vi "Thermal Waveforms.vi"(10 "Log Read Data":cluster{refnum<class "RDS State.lvclass">[]}[](array[cluster]), 11 "Header":T1) -> (2 "Log Data Out":cluster{refnum<class "RDS State.lvclass">[]}[](array[cluster]), 3 "Header Out":T1, 5 "Thermal WFs":waveform(dbl)[](array[waveform]))   [LabVIEW 2015, in "Log Waveform Processors.lvlib"]
uses:
  Log Waveform Processors.lvlib
  RDS State Tracker/RDS State/RDS State.lvclass
  Actors/RDS Logger Actor/RDS Logger Actor/RDS Logger Actor/Logger Header.ctl
  RDS State Tracker/RDS State/RDS State.lvclass/RDS State.ctl
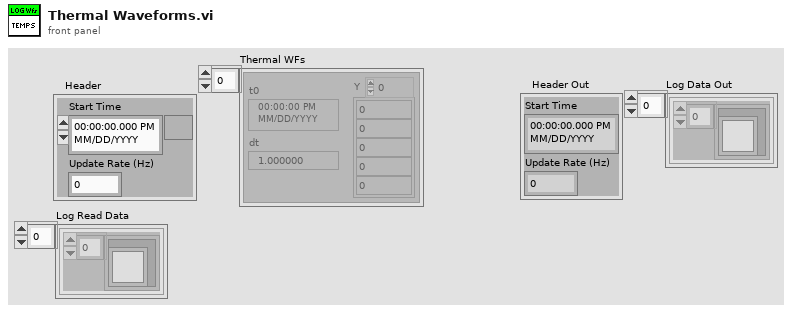
[diagram p1: front panel]
types:
  T1 = typedef "Log Waveform Processors.lvlib/Logger Header.ctl" = cluster{"Start Time":timestamp, "Update Rate (Hz)":dbl}
  T2 = typedef "RDS Instrument Library.lvlib/Battery Data.ctl" = cluster{"Battery Status":T3, "Pack Voltage":sgl, "Pack Current":sgl, "Pack Capacity":sgl, "Max Cell Temp":sgl, "Min Cell Temp":sgl, "Max Cell Voltage":sgl, "Min Cell Voltage":sgl}
  T3 = typedef "RDS Instrument Library.lvlib/Battery Status.ctl" = enum16{"Pack Normal", "Alarm: Cell temp too high", "Alarm: Pack voltage too high", "Warn: Pack voltage too high ", "Alarm: Pack voltage too low", "Warn: Pack voltage low", "Alarm Pack current too high", "Warn: Pack current too high ", "Fault: Pack to chassis connection detected", "Fault: Pack to cell connection error", "Fautl: System error"}
  T4 = typedef "RDS Instrument Library.lvlib/Compass Data.ctl" = cluster{"Compass Heading":sgl, "pitch Angle":sgl, "roll Angle":sgl, "Temperature":sgl, "Depth":sgl, "Magnetic Field":sgl, "Magnetic Field X":sgl, "Magnetic Field Y":sgl, "Magnetic Field Z":sgl, "Acceleration":sgl, "Acceleration X":sgl, "Acceleration Y":sgl, "Gyro":sgl, "Gyro X":sgl, "Acceleration Z":sgl, "Gyro Y":sgl, "Raw Heading":sgl}
  T5 = typedef "RDS Child Messages.lvlib/MCB Motor Status.ctl" = cluster{"Motor Power":i16, "Motor Command":i16, "Battery Volts":sgl, "Battery Amps":sgl, "Motor Amps":sgl, "MCU Temp":i16, "Heatsink Temp":i16, "Fault Flags":u16, "StatusFlags":u16}
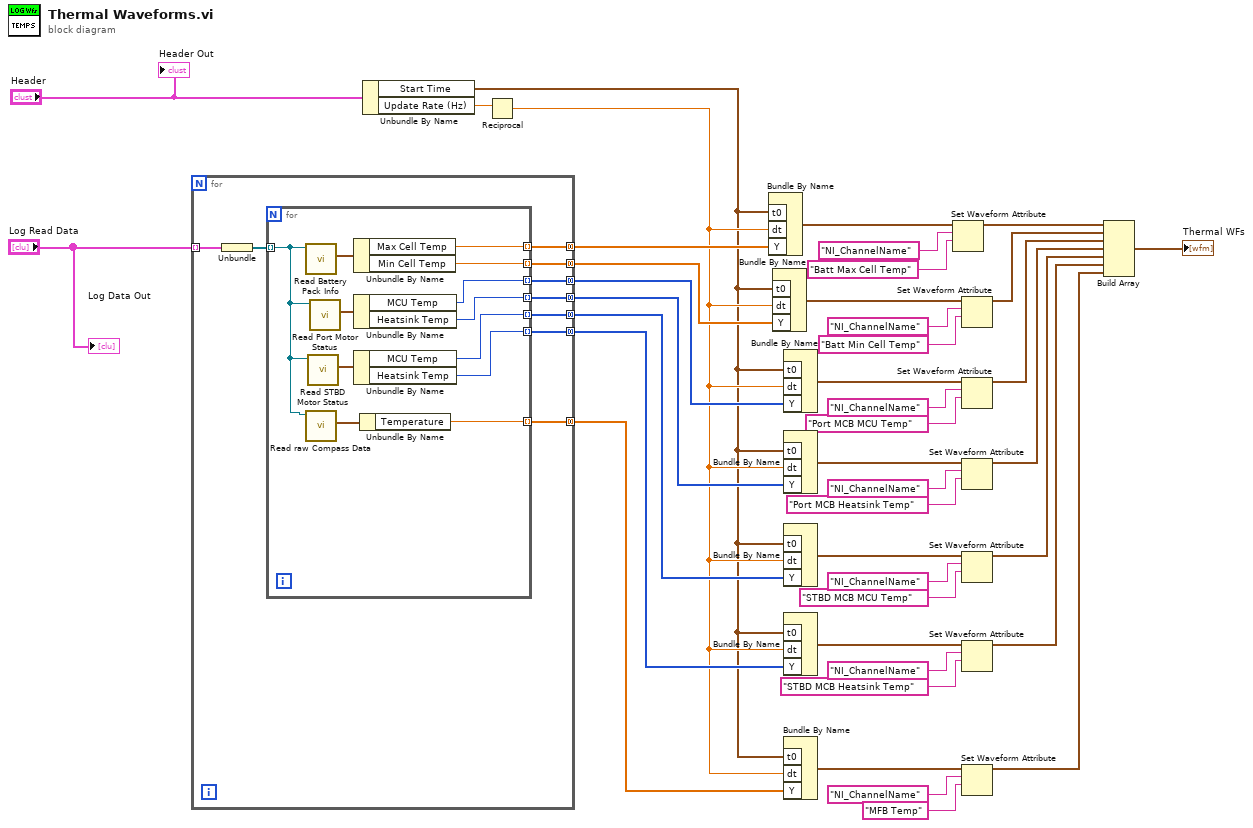
[diagram p0: block diagram]
diagram:
  n1 = for {
    tunnel: "Log Read Data" -> [w50] mode=indexing
    tunnel: [w48] -> w12 mode=concatenating
    tunnel: [w47] -> w17 mode=concatenating
    tunnel: [w46] -> w18 mode=concatenating
    tunnel: [w45] -> w34 mode=concatenating
    tunnel: [w44] -> w35 mode=concatenating
    tunnel: [w43] -> w38 mode=concatenating
    tunnel: [w42] -> w4 mode=concatenating
    n2 = Unbundle(w50) -> (w49:refnum<class "RDS State.lvclass">[])
    n3 = for {
      tunnel: w49 -> [w53] mode=indexing
      tunnel: [w61] -> w48 mode=indexing
      tunnel: [w60] -> w47 mode=indexing
      tunnel: [w57] -> w46 mode=indexing
      tunnel: [w56] -> w45 mode=indexing
      tunnel: [w55] -> w44 mode=indexing
      tunnel: [w54] -> w43 mode=indexing
      tunnel: [w51] -> w42 mode=indexing
      n4 = call "Read Battery Pack Info.vi"("RDS State in"=w53) -> ("Battery Pack Info"=w62:T2)  [unwired: 8 in, 2 out]
      n5 = call "Read raw Compass Data.vi"("RDS State in"=w53) -> ("Compass Data"=w52:T4)  [unwired: 8 in, 2 out]
      n6 = call "Read STBD Motor Status.vi"("RDS State in"=w53) -> ("STBD Motor"=w58:T5)  [unwired: 8 in, 2 out]
      n7 = call "Read Port Motor Status.vi"("RDS State in"=w53) -> ("Port Motor Data"=w59:T5)  [unwired: 8 in, 2 out]
      n8 = Unbundle By Name(w62) -> ("Max Cell Temp"=w61:sgl, "Min Cell Temp"=w60:sgl)
      n9 = Unbundle By Name(w59) -> ("MCU Temp"=w57:i16, "Heatsink Temp"=w56:i16)
      n10 = Unbundle By Name(w58) -> ("MCU Temp"=w55:i16, "Heatsink Temp"=w54:i16)
      n11 = Unbundle By Name(w52) -> ("Temperature"=w51:sgl)
    }
  }
  n12 = Unbundle By Name("Header") -> ("Start Time"=w2:timestamp, "Update Rate (Hz)"=w9:dbl)
  n13 = Reciprocal(x=w9) -> (1/x=w3:dbl)
  n14 = Bundle By Name("t0"=w2, "dt"=w3, "Y"=w12) -> (w13:waveform(sgl))  [unwired: 1 in]
  n15 = Bundle By Name("t0"=w2, "dt"=w3, "Y"=w17) -> (w15:waveform(sgl))  [unwired: 1 in]
  n16 = Bundle By Name("t0"=w2, "dt"=w3, "Y"=w18) -> (w16:waveform(i16))  [unwired: 1 in]
  n17 = Bundle By Name("t0"=w2, "dt"=w3, "Y"=w34) -> (w30:waveform(i16))  [unwired: 1 in]
  n18 = Bundle By Name("t0"=w2, "dt"=w3, "Y"=w35) -> (w31:waveform(i16))  [unwired: 1 in]
  n19 = Bundle By Name("t0"=w2, "dt"=w3, "Y"=w38) -> (w37:waveform(i16))  [unwired: 1 in]
  n20 = Bundle By Name("t0"=w2, "dt"=w3, "Y"=w4) -> (w5:waveform(sgl))  [unwired: 1 in]
  n21 = Set Waveform Attribute(5:"Batt Max Cell Temp" ("name"), 6:"NI_ChannelName" ("name"), 7:w13) -> (3:w19:waveform(sgl))  [unwired: 1 in, 2 out]
  n22 = Set Waveform Attribute(5:"Batt Min Cell Temp" ("name"), 6:"NI_ChannelName" ("name"), 7:w15) -> (3:w20:waveform(sgl))  [unwired: 1 in, 2 out]
  n23 = Set Waveform Attribute(5:"Port MCB MCU Temp" ("name"), 6:"NI_ChannelName" ("name"), 7:w16) -> (3:w21:waveform(i16))  [unwired: 1 in, 2 out]
  n24 = Set Waveform Attribute(5:"Port MCB Heatsink Temp" ("name"), 6:"NI_ChannelName" ("name"), 7:w30) -> (3:w39:waveform(i16))  [unwired: 1 in, 2 out]
  n25 = Set Waveform Attribute(5:"STBD MCB MCU Temp" ("name"), 6:"NI_ChannelName" ("name"), 7:w31) -> (3:w40:waveform(i16))  [unwired: 1 in, 2 out]
  n26 = Set Waveform Attribute(5:"STBD MCB Heatsink Temp" ("name"), 6:"NI_ChannelName" ("name"), 7:w37) -> (3:w41:waveform(i16))  [unwired: 1 in, 2 out]
  n27 = Set Waveform Attribute(5:"MFB Temp" ("name"), 6:"NI_ChannelName" ("name"), 7:w5) -> (3:w1:waveform(sgl))  [unwired: 1 in, 2 out]
  n28 = Build Array(w19, w20, w21, w39, w40, w41, w1) -> (→"Thermal WFs":waveform(sgl)[])
  "Header Out" <- "Header"
  "Log Data Out" <- "Log Read Data"
